vi "Check Status (No Objects) - Laser power controller.vi"(8 "error in (no error)":errorcluster, 10 "VISA Resource Name":refnum<visa-resource-name>="GPIB0::3::INSTR", 11 "Cluster In":T1) -> (0 "error out":errorcluster, 1 "Status":string, 2 "Ready?":bool, 3 "Cluster Out":T1)   [LabVIEW 2012]
doc: "(Dynamic) Check if the instrument is powered on and update its member fields with the instrument's current status. Optionally return a text status message."
uses:
  BEOC LPC/BEOC LPC.lvlib
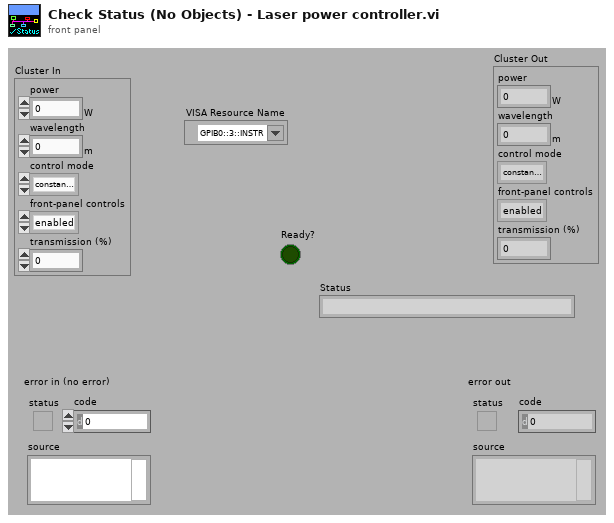
[diagram p1: front panel]
types:
  T1 = cluster{"power":dbl[unit], "wavelength":dbl[unit], "control mode":enum16{"constant power", "constant transmission"}, "front-panel controls":enum16{"enabled", "disabled"}, "transmission (%)":dbl}
  T2 = enum16{"constant power", "constant transmission"}
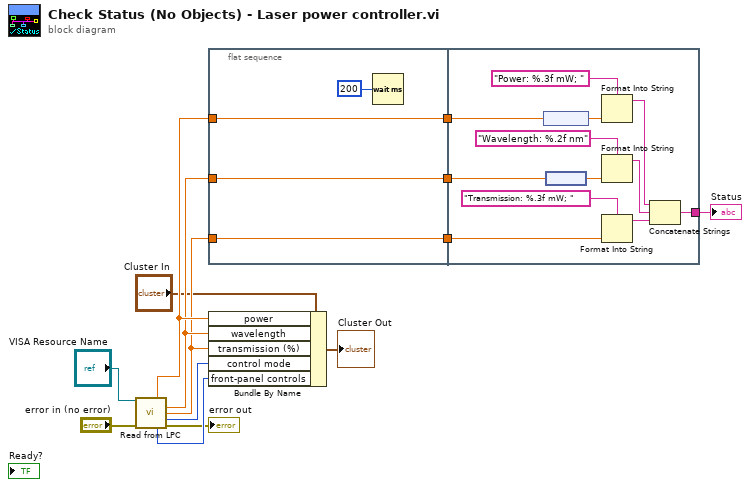
[diagram p0: block diagram]
diagram:
  n1 = call "Read from LPC.vi"("VISA resource name"="VISA Resource Name", "error in (no error)"="error in (no error)") -> ("power"=w12:dbl[unit], "wavelength"=w11:dbl[unit], "Transmission"=w9:dbl, "control mode"=w14:T2, "front-panel controls"=w13:enum16{"enabled", "disabled"}, "error out"=→"error out":errorcluster)  [unwired: 7 in, 1 out]
  n2 = flat-sequence {
    tunnel: w9 -> [w16]
    tunnel: w11 -> [w17]
    tunnel: w12 -> [w18]
    tunnel: [w18] -> w8
    tunnel: [w17] -> w7
    tunnel: [w16] -> w6
    tunnel: [w24] -> w10
    tunnel: w8 -> [w30]
    tunnel: w7 -> [w28]
    tunnel: w6 -> [w19]
    frame #0 {
      n3 = Wait (ms)(milliseconds to wait=u32 200) -> ()  [unwired: 1 out]
    }
    frame #1 {
      n4 = node(w30) -> (w23:dbl)
      n5 = node(w28) -> (w22:dbl)
      n6 = Format Into String(format string="Power: %.3f mW; ", w23) -> (resulting string=w25:string)  [unwired: 2 in, 1 out]
      n7 = Format Into String(format string="Wavelength: %.2f nm", w22) -> (resulting string=w26:string)  [unwired: 2 in, 1 out]
      n8 = Format Into String(format string="Transmission: %.3f mW; ", w19) -> (resulting string=w20:string)  [unwired: 2 in, 1 out]
      n9 = Concatenate Strings(w25, w26, w20) -> (w24:string)
    }
  }
  n10 = Bundle By Name(cluster="Cluster In", "power"=w12, "wavelength"=w11, "transmission (%)"=w9, "control mode"=w14, "front-panel controls"=w13) -> (→"Cluster Out":T1)
  "Status" <- w10
